vi "MotorControl.vi"(8 "error in":errorcluster, 10 "ValueIn":T1, 11 "Reference In":T2={"VISA resource name"="", "MotorType"=enum."AK80-64", "CAN ID"=1}) -> (0 "error out":errorcluster, 2 "FilteredValue":T1, 3 "Reference Out":T2={"VISA resource name"="", "MotorType"=enum."AK80-64", "CAN ID"=1})   [LabVIEW 2019, in "CubeMarsBLDClib.lvlib"]
uses:
  CubeMarsBLDClib.lvlib
  Reference.ctl
  MotorType.ctl
  MotorParameters.ctl
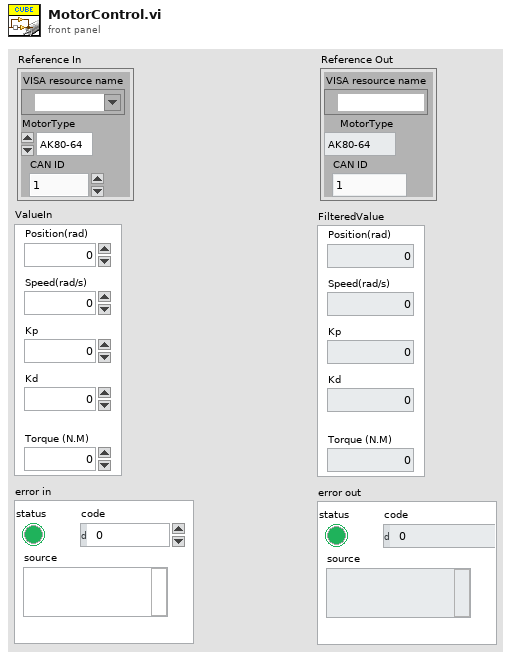
[diagram p1: front panel]
types:
  T1 = typedef "CubeMarsBLDClib.lvlib/MotorParameters.ctl" = cluster{"Position(rad)":dbl, "Speed(rad/s)":dbl, "Kp":dbl, "Kd":dbl, "Torque (N.M)":dbl}
  T2 = typedef "CubeMarsBLDClib.lvlib/Reference.ctl" = cluster{"VISA resource name":refnum<visa-resource-name>, "MotorType":T3, "CAN ID":u32}
  T3 = typedef "CubeMarsBLDClib.lvlib/MotorType.ctl" = enum16{"AK80-64", "AK80-9", "AK80-8", "AK80-6", "AK70-10", "AK60-6", "AK10-9"}
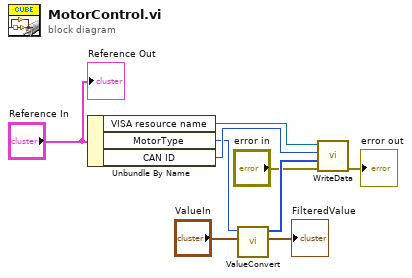
[diagram p0: block diagram]
diagram:
  n1 = Unbundle By Name("Reference In") -> ("VISA resource name"=w9:refnum<visa-resource-name>, "MotorType"=w7:T3, "CAN ID"=w8:u32)
  n2 = call "ValueConvert.vi"("ValueIn"="ValueIn", "MotorType"=w7) -> ("FilteredValue"=→"FilteredValue":T1, "CANBusData"=w5:u8[])  [unwired: 8 in]
  n3 = call "WriteData.vi"("error in"="error in", "Data(0~8Byte)"=w5, "ID"=w8, "VISA Refnum in"=w9) -> ("error out"=→"error out":errorcluster)  [unwired: 6 in, 1 out]
  "Reference Out" <- "Reference In"
